vi "setFreq.vi"(3 "error in":errorcluster, 5 "Frequenz in Hz":dbl=200.0 format="%.2f") -> (0 "error out":errorcluster)   [LabVIEW 2010]
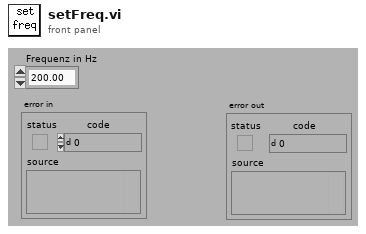
[diagram p1: front panel]
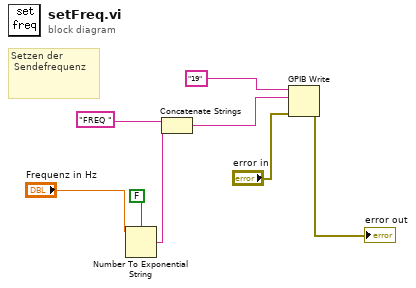
[diagram p0: block diagram]
diagram:
  # "Setzen der \n Sendefrequenz"
  n1 = Number To Exponential String(number="Frequenz in Hz", 1:FALSE ("use system decimal point (T)")) -> (E-format string=w3:string)  [unwired: 2 in]
  n2 = Concatenate Strings("FREQ ", w3) -> (w1:string)
  n3 = GPIB Write(0:"19", 1:w1, 3:"error in") -> (6:→"error out":errorcluster)  [unwired: 2 in, 1 out]
